vi "to json.vi"(8 "error in":errorcluster, 10 "dataSourceRid":string, 11 "stream_custom_cluster in":refnum<class "stream_custom_cluster.lvclass">) -> (0 "error out":errorcluster, 1 "Contains Data":bool, 2 "json":string, 3 "stream_custom_cluster out":refnum<class "stream_custom_cluster.lvclass">, 4 "Terminated":bool)   [LabVIEW 2020, in "stream_custom_cluster.lvclass"]
uses:
  stream_custom_cluster.lvclass
  stream_custom_cluster.lvclass/stream_custom_cluster.ctl
  50db6b1e-7037-4d0a-8807-b72f8bc667cd.vi
  3d1b79a7-f0f8-4911-8cd0-6b30bac1e9f1.vi
  d27922d7-2c6b-4151-838e-76c4f3329ecb.vi
  <vilib>/JDP Science/JSONtext/Variant to JSON Text.vi
  <vilib>/JDP Science/JSONtext/support/Format JSON Array Text.vi
  <vilib>/JDP Science/JSONtext/LVClass Serializer/JSONtext LVClass Serializer.lvclass
  <vilib>/JDP Science/JSONtext/JSONtext.lvlib
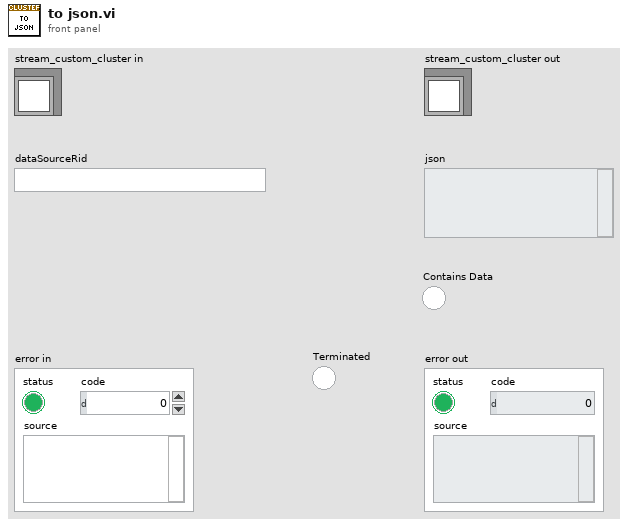
[diagram p1: front panel]
types:
  T1 = typedef "openg_variant.lvlib/Type Descriptor Enumeration__ogtk.ctl" = enum8{"<Null>", "I8", "I16", "I32", "I64", "U8", "U16", "U32", "U64", "SGL", "DBL", "EXT", "CSG", "CDB", "CXT", "0x0F", "0x10", "0x11", "0x12", "0x13", "0x14", "Enum U8", "Enum U16", "Enum U32", "Enum U64", "SGL PQ", "DBL PQ", "EXT PQ", "CSG PQ", "CDB PQ", "CXT PQ", "0x1F", "0x20", "Boolean", "0x22", "0x23", "0x24", "0x25", "0x26", "0x27", "0x28", "0x29", "0x2A", "0x2B", "0x2C", "0x2D", "0x2E", "0x2F", "String", "0x31", "Path", "Pict", "0x34", "0x35", "0x36", "DAQ", "0x38", "0x39", "0x3A", "0x3B", "0x3C", "0x3D", "0x3E", "0x3F", "Array", "0x41", "0x42", "0x43", "0x44", "0x45", "0x46", "0x47", "0x48", "0x49", "0x4A", "0x4B", "0x4C", "0x4D", "0x4E", "0x4F", "Cluster", "0x51", "0x52", "Variant", "Waveform", "0x55", "0x56", "0x57", "0x58", "0x59", "0x5A", "0x5B", "0x5C", "0x5D", "0x5E", "Fixed Point", "0x60", "0x61", "0x62", "0x63", "0x64", "0x65", "0x66", "0x67", "0x68", "0x69", "0x6A", "0x6B", "0x6C", "0x6D", "0x6E", "0x6F", "Refnum", "0x71", "0x72", "Set Collection", "Map Collection"}
  T2 = cluster{"type":T1[], "channel names":string[], "data":refnum<queue>[]}
  T3 = cluster{"timestamp":cluster{"seconds":i32, "nanos":i32}, "value":variant}[]
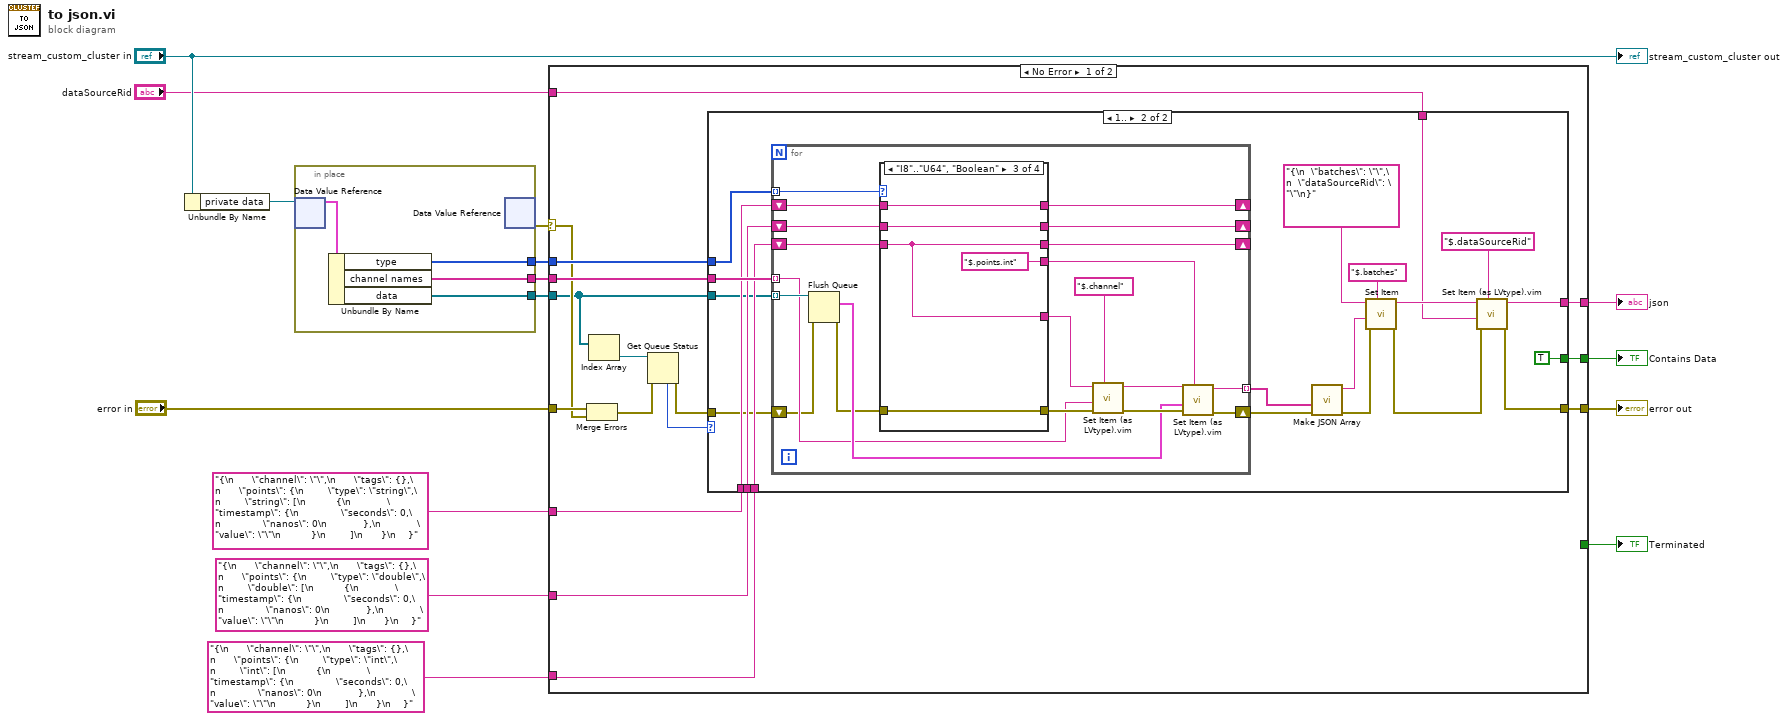
[diagram p0: block diagram]
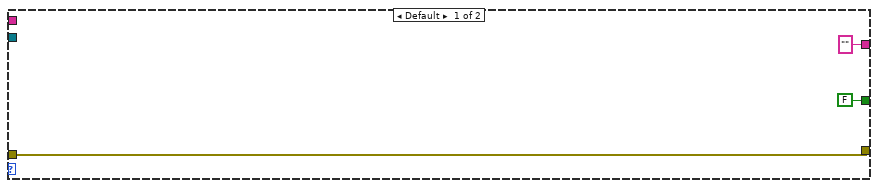
[diagram p2: hidden frame]
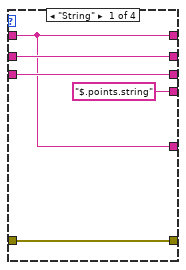
[diagram p3: hidden frame]
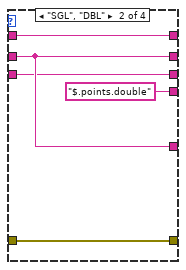
[diagram p4: hidden frame]
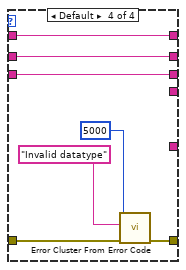
[diagram p5: hidden frame]
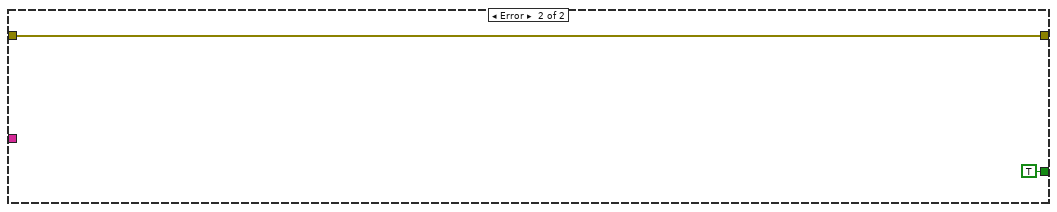
[diagram p6: hidden frame]
diagram:
  n1 = Unbundle By Name("stream_custom_cluster in") -> ("private data"=w14:refnum<data-value>)
  n2 = in-place {
    in-place-border: [w16] -> w3
    in-place-border: [w18] -> w13
    in-place-border: [w17] -> w12
    n3 = in-place-dvr #1(w14) -> (w19:T2)  [unwired: 1 out]
    n4 = Unbundle By Name(w19) -> ("type"=w17:T1[], "channel names"=w18:string[], "data"=w16:refnum<queue>[])
    n5 = in-place-dvr #1() -> (w4:errorcluster)  [unwired: 1 in, 1 out]
  }
  n6 = case shown="No Error" w4 {
    selector: w4 -> [w26 _]
    tunnel: w13 -> [w35 _]
    tunnel: w12 -> [w34 _]
    tunnel: "{\n      \"channel\": \"\",\n      \"tags\": {},\n      \"points\": {\n        \"type\": \"string\",\n        \"string\": [\n          {\n            \"timestamp\": {\n              \"seconds\": 0,\n              \"nanos\": 0\n            },\n            \"value\": \"\"\n          }\n        ]\n      }\n    }" ("String") -> [w33 _]
    tunnel: "{\n      \"channel\": \"\",\n      \"tags\": {},\n      \"points\": {\n        \"type\": \"double\",\n        \"double\": [\n          {\n            \"timestamp\": {\n              \"seconds\": 0,\n              \"nanos\": 0\n            },\n            \"value\": \"\"\n          }\n        ]\n      }\n    }" ("String") -> [w32 _]
    tunnel: "{\n      \"channel\": \"\",\n      \"tags\": {},\n      \"points\": {\n        \"type\": \"int\",\n        \"int\": [\n          {\n            \"timestamp\": {\n              \"seconds\": 0,\n              \"nanos\": 0\n            },\n            \"value\": \"\"\n          }\n        ]\n      }\n    }" ("String") -> [w31 _]
    tunnel: [w30 w102] -> w8
    tunnel: "dataSourceRid" -> [w29 _]
    tunnel: [w28 _] -> w6
    tunnel: "error in" -> [w27 w102]
    tunnel: w3 -> [w25 _]
    tunnel: [w20 _] -> w2
    tunnel: [_ TRUE] -> w1
    frame No Error {
      n7 = Merge Errors(w27, w26) -> (w23:errorcluster)
      n8 = Index Array(array=w25) -> (element=w24:refnum<queue>)  [unwired: 1 in]
      n9 = Get Queue Status(queue=w24, error in (no error)=w23) -> (error out=w22:errorcluster, # elements in queue=w21:i32)  [unwired: 1 in, 6 out]
      n10 = case shown="1.." w21 {
        tunnel: w35 -> [_ w58]
        tunnel: w34 -> [_ w57]
        tunnel: w33 -> [_ w56]
        tunnel: w32 -> [_ w55]
        tunnel: w31 -> [_ w54]
        tunnel: [w38 w44] -> w30
        tunnel: w29 -> [_ w43]
        tunnel: ["" ("<JSON>") w42] -> w28
        tunnel: w25 -> [_ w41]
        tunnel: w22 -> [w38 w40]
        tunnel: [FALSE TRUE] -> w20
        frame Default {
        }
        frame 1.. {
          n11 = for {
            tunnel: w57 -> [w64] mode=indexing
            shift-right: [w73] -> _
            shift-left: w56 -> [w76]
            shift-right: [w72] -> _
            shift-left: w55 -> [w75]
            shift-right: [w71] -> _
            shift-left: w54 -> [w74]
            tunnel: [w66] -> w46 mode=indexing
            shift-right: [w65] -> w45
            shift-left: w40 -> [w59]
            tunnel: w41 -> [w63] mode=indexing
            tunnel: w58 -> [w61] mode=indexing
            n12 = Flush Queue(queue=w63, error in (no error)=w59) -> (remaining elements=w62:T3, error out=w60:errorcluster)  [unwired: 1 out]
            n13 = case shown="\"I8\"..\"U64\", \"Boolean\"" w64 {
              tunnel: w60 -> [w83 w88 w93 w96]
              tunnel: [w83 w88 w93 w97] -> w77
              tunnel: w76 -> [w80 w86 w91 w100]
              tunnel: w75 -> [w81 w87 w90 w99]
              tunnel: w74 -> [w82 w85 w92 w98]
              tunnel: [w80 w86 w91 w100] -> w73
              tunnel: [w81 w87 w90 w99] -> w72
              tunnel: [w82 w85 w92 w98] -> w71
              tunnel: [w80 w87 w92 _] -> w70
              tunnel: ["$.points.string" ("$Path or Item Name") "$.points.double" ("$Path or Item Name") "$.points.int" ("$Path or Item Name") _] -> w67
              frame "String" {
              }
              frame "SGL", "DBL" {
              }
              frame "I8".."U64", "Boolean" {
              }
              frame Default {
                n14 = call <vilib>:"Error Cluster From Error Code.vi"("error in (no error)"=w96, "error message (\"\")"="Invalid datatype" ("error message (\"\")"), "error code (0)"=5000) -> ("error out"=w97:errorcluster)  [unwired: 6 in]
              }
            }
            n15 = call "Set Item (as LVtype).vim"("$Path or Item Name"="$.channel", "error in (no error)"=w77, "Anything"=w61, "JSON"=w70) -> ("error out"=w68:errorcluster, "<JSON>"=w69:string)  [unwired: 4 in, 1 out]
            n16 = call "Set Item (as LVtype).vim"("$Path or Item Name"=w67, "error in (no error)"=w68, "Anything"=w62, "JSON"=w69) -> ("error out"=w65:errorcluster, "<JSON>"=w66:string)  [unwired: 4 in, 1 out]
          }
          n17 = call <vilib>:"Make JSON Array.vi"("error in (no error)"=w45, "JSON Elements"=w46) -> ("error out"=w47:errorcluster, "<JSON>"=w52:string)  [unwired: 8 in]
          n18 = call <vilib>:"Set Item.vi"("$Path or Item Name"="$.batches", "error in (no error)"=w47, "JSON to Insert"=w52, "JSON"="{\n  \"batches\": \"\",\n  \"dataSourceRid\": \"\"\n}") -> ("error out"=w48:errorcluster, "<JSON>"=w49:string)  [unwired: 4 in, 1 out]
          n19 = call "Set Item (as LVtype).vim"("$Path or Item Name"="$.dataSourceRid", "error in (no error)"=w48, "Anything"=w43, "JSON"=w49) -> ("error out"=w44:errorcluster, "<JSON>"=w42:string)  [unwired: 4 in, 1 out]
        }
      }
    }
    frame Error {
    }
  }
  "error out" <- w8
  "json" <- w6
  "Contains Data" <- w2
  "Terminated" <- w1
  "stream_custom_cluster out" <- "stream_custom_cluster in"
